vi "Init.vi"(7 "I2C Options":T2={"Bus"=0, "Baud"=400000, "SCL GPIO"=16, "SDA GPIO"=17}, 8 "error in (no error)":errorcluster, 9 "LCD Size":T1={"Rows"=2, "Cols"=16}, 10 "VISA resource name in":refnum<visa-resource-name>, 11 "Address":u8=39 format="%.0x") -> (0 "error out":errorcluster, 2 "VISA resource name":refnum<visa-resource-name>, 3 "LCD-I2C out":refnum<class "LCD-I2C.lvclass">)   [LabVIEW 2023, in "CTI-Visa-DeviceLib.lvlib" / "LCD-I2C.lvclass"]
uses:
  LCD-I2C.lvclass
  CTI-Visa/I2C Options.ctl
  LCD Size.ctl
  CTI-Visa/Digital Pull Direction.ctl
  LCD-I2C.lvclass/LCD-I2C.ctl
  CTI-Visa/CTI-Visa.lvlib
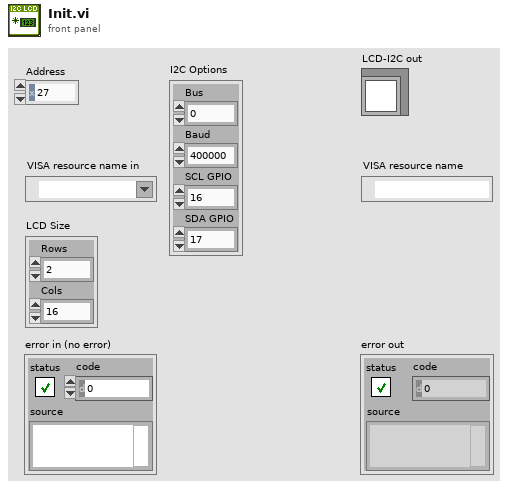
[diagram p1: front panel]
types:
  T1 = typedef "CTI-Visa-DeviceLib.lvlib/LCD-I2C.lvclass/LCD Size.ctl" = cluster{"Rows":u8, "Cols":u8}
  T2 = typedef "CTI-Visa.lvlib/I2C Options.ctl" = cluster{"Bus":u8, "Baud":u32, "SCL GPIO":i32, "SDA GPIO":i32}
  T3 = typedef "CTI-Visa.lvlib/Digital Pull Direction.ctl" = enum16{"None", "Up", "Down", "Both"}
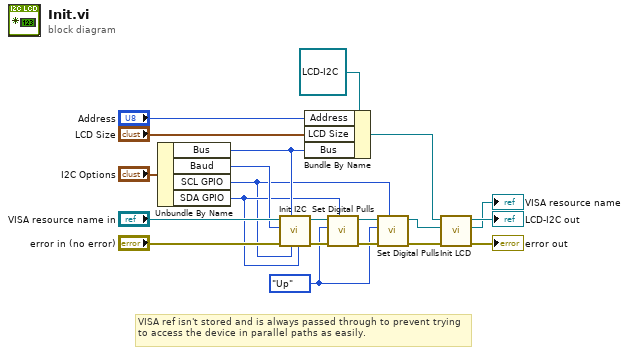
[diagram p0: block diagram]
diagram:
  w3 = Digital_Pull_Direction."Up" ("Pull")
  # "VISA ref isn't stored and is always passed through to prevent trying to access the device in parallel paths as easily."
  n1 = Unbundle By Name("I2C Options") -> ("Bus"=w11:u8, "Baud"=w10:u32, "SCL GPIO"=w4:i32, "SDA GPIO"=w7:i32)
  n2 = call "Init I2C.vi"("SDA GPIO"=w7, "SCL GPIO"=w4, "Bus"=w11, "error in (no error)"="error in (no error)", "Baud"=w10, "VISA resource name in"="VISA resource name in") -> ("error out"=w9:errorcluster, "VISA resource name"=w8:refnum<visa-resource-name>)  [unwired: 4 in]
  n3 = Bundle By Name(cluster=refnum<class "LCD-I2C.lvclass"> refnum ("LCD-I2C in"), "Address"="Address", "LCD Size"="LCD Size", "Bus"=w11) -> (w17:refnum<class "LCD-I2C.lvclass">)
  n4 = call "Set Digital Pulls.vi"("GPIO"=w7, "error in (no error)"=w9, "Pull"=w3, "VISA resource name in"=w8) -> ("error out"=w6:errorcluster, "VISA resource name"=w5:refnum<visa-resource-name>)  [unwired: 6 in]
  n5 = call "Set Digital Pulls.vi"("GPIO"=w4, "error in (no error)"=w6, "Pull"=w3, "VISA resource name in"=w5) -> ("error out"=w2:errorcluster, "VISA resource name"=w1:refnum<visa-resource-name>)  [unwired: 6 in]
  n6 = call "Init LCD.vi"("error in (no error)"=w2, "VISA resource name in"=w1, "LCD-I2C in"=w17) -> ("error out"=→"error out":errorcluster, "VISA resource name"=→"VISA resource name":refnum<visa-resource-name>, "LCD-I2C out"=→"LCD-I2C out":refnum<class "LCD-I2C.lvclass">)  [unwired: 6 in]
